vi "SCTL Sector Accumulation.vi"() -> (2 "Accummulated":T1(array[cluster]), 3 "New Data?":bool)   [LabVIEW 2013]
uses:
  Accumulated Count Array Fixed Point.ctl
  <vilib>/rvi/FIFO/Fifo_Resource/nirvififoEmulationReadFpgaImpl.vi
  <vilib>/rvi/DataTransferAndStorage/Container/Common/niFpgaContainerGetUniqueNameForEmu.vi
  <vilib>/rvi/Memory/Memory_Emulation/nirvimemoryFastEmulationFpgaImpl.vi
  <instcachedir>/0/nirvimemoryFastEmulationFpgaImpl_5FBAB50466BC4C939F684F8805638BFC.lvgen/nirvimemoryFastEmulationFpgaImpl_5FBAB50466BC4C939F684F8805638BFC_012.vi
  <vilib>/rvi/Memory/Memory_Emulation/nirvimemoryFastEmulation.vi
  <vilib>/rvi/Memory/Memory_Emulation/nirvimemoryEmulation.vi
  <vilib>/rvi/DataTransferAndStorage/Container/XNode/niFpgaContainer.xnode
  <vilib>/rvi/FIFO/Fifo_Resource/nirvififoEmulationRead.vi
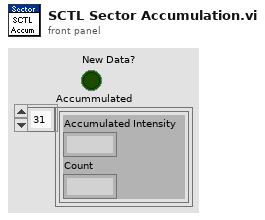
[diagram p1: front panel]
types:
  T1 = cluster{"Accumulated Intensity":fxp<+,20,20>, "Count":fxp<+,12,12>}[]
  T2 = cluster{"Accumulated Intensity":fxp<+,8,8>, "Count":fxp<+,1,1>}
  T3 = typedef "Accumulated Count Array Fixed Point.ctl" = cluster{"Accumulated Intensity":fxp<+,20,20>, "Count":fxp<+,12,12>}[]
  T4 = cluster{"Accumulated Intensity":fxp<+,21,21>, "Count":fxp<+,13,13>}[]
  T5 = cluster{"Accumulated Intensity":fxp<+,22,22>, "Count":fxp<+,14,14>}[]
  T6 = cluster{"Accumulated Intensity":fxp<+,23,23>, "Count":fxp<+,15,15>}[]
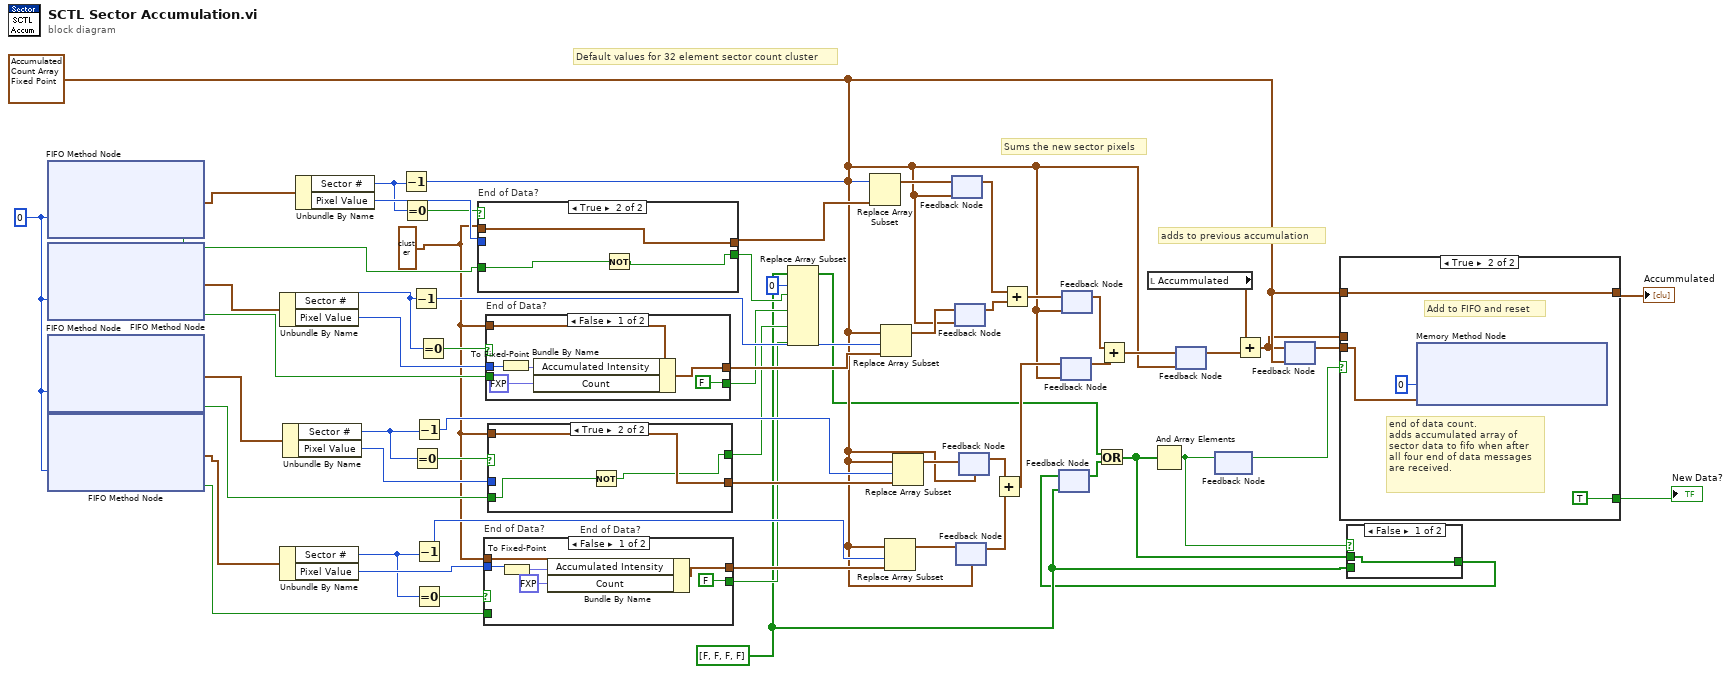
[diagram p0: block diagram]
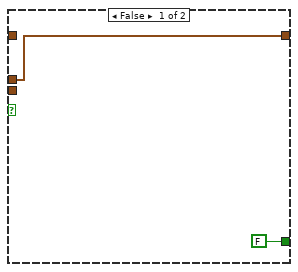
[diagram p3: hidden frame]
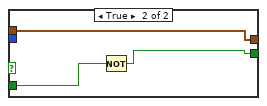
[diagram p4: hidden frame]
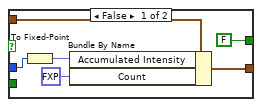
[diagram p5: hidden frame]
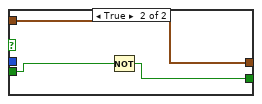
[diagram p6: hidden frame]
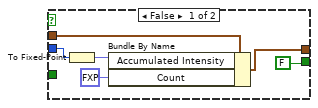
[diagram p7: hidden frame]
diagram:
  w5 = 0 ("Timeout")
  w7 = bool[] [FALSE, FALSE, FALSE, FALSE]
  w37 = T2 {"Accumulated Intensity"=0.0, "Count"=0.0} ("Accumulated Sector Cluster")
  w19 = T3 [{"Accumulated Intensity"=0.0, "Count"=0.0}, {"Accumulated Intensity"=0.0, "Count"=0.0}, {"Accumulated Intensity"=0.0, "Count"=0.0}, {"Accumulated Intensity"=0.0, "Count"=0.0}, {"Accumulated Intensity"=0.0, "Count"=0.0}, {"Accumulated Intensity"=0.0, "Count"=0.0}, {"Accumulated Intensity"=0.0, "Count"=0.0}, {"Accumulated Intensity"=0.0, "Count"=0.0}, {"Accumulated Intensity"=0.0, "Count"=0.0}, {"Accumulated Intensity"=0.0, "Count"=0.0}, {"Accumulated Intensity"=0.0, "Count"=0.0}, {"Accumulated Intensity"=0.0, "Count"=0.0}, {"Accumulated Intensity"=0.0, "Count"=0.0}, {"Accumulated Intensity"=0.0, "Count"=0.0}, {"Accumulated Intensity"=0.0, "Count"=0.0}, {"Accumulated Intensity"=0.0, "Count"=0.0}, {"Accumulated Intensity"=0.0, "Count"=0.0}, {"Accumulated Intensity"=0.0, "Count"=0.0}, {"Accumulated Intensity"=0.0, "Count"=0.0}, {"Accumulated Intensity"=0.0, "Count"=0.0}, {"Accumulated Intensity"=0.0, "Count"=0.0}, {"Accumulated Intensity"=0.0, "Count"=0.0}, {"Accumulated Intensity"=0.0, "Count"=0.0}, {"Accumulated Intensity"=0.0, "Count"=0.0}, {"Accumulated Intensity"=0.0, "Count"=0.0}, {"Accumulated Intensity"=0.0, "Count"=0.0}, {"Accumulated Intensity"=0.0, "Count"=0.0}, {"Accumulated Intensity"=0.0, "Count"=0.0}, {"Accumulated Intensity"=0.0, "Count"=0.0}, {"Accumulated Intensity"=0.0, "Count"=0.0}, {"Accumulated Intensity"=0.0, "Count"=0.0}, {"Accumulated Intensity"=0.0, "Count"=0.0}] ("Test Accumulated Array")
  # "adds to previous accumulation"
  # "Sums the new sector pixels"
  # "Default values for 32 element sector count cluster"
  n1 = xnode ("FIFO Method Node")("Timeout"=w5) -> ("Element"=w4:cluster{"Sector #":u8, "Pixel Value":u8}, "Timed Out?"=w41:bool)  [unwired: 1 in, 1 out]
  n2 = xnode ("FIFO Method Node")("Timeout"=w5) -> ("Element"=w3:cluster{"Sector #":u8, "Pixel Value":u8}, "Timed Out?"=w40:bool)  [unwired: 1 in, 1 out]
  n3 = xnode ("FIFO Method Node")("Timeout"=w5) -> ("Element"=w2:cluster{"Sector #":u8, "Pixel Value":u8}, "Timed Out?"=w39:bool)  [unwired: 1 in, 1 out]
  n4 = xnode ("FIFO Method Node")("Timeout"=w5) -> ("Element"=w1:cluster{"Sector #":u8, "Pixel Value":u8}, "Timed Out?"=w38:bool)  [unwired: 1 in, 1 out]
  n5 = Unbundle By Name(w3) -> ("Sector #"=w49:u8, "Pixel Value"=w59:u8)
  n6 = Unbundle By Name(w1) -> ("Sector #"=w45:u8, "Pixel Value"=w53:u8)
  n7 = Unbundle By Name(w2) -> ("Sector #"=w47:u8, "Pixel Value"=w56:u8)
  n8 = Unbundle By Name(w4) -> ("Sector #"=w51:u8, "Pixel Value"=w61:u8)
  n9 = Decrement(x=w51) -> (x-1=w62:u8)
  n10 = Equal To 0?(x=w51) -> (x = 0?=w50:bool)
  n11 = Decrement(x=w49) -> (x-1=w58:u8)
  n12 = Equal To 0?(x=w47) -> (x = 0?=w46:bool)
  n13 = Decrement(x=w47) -> (x-1=w42:u8)
  n14 = Decrement(x=w45) -> (x-1=w55:u8)
  n15 = Equal To 0?(x=w45) -> (x = 0?=w44:bool)
  n16 = Equal To 0?(x=w49) -> (x = 0?=w48:bool)
  n17 = case "End of Data?" shown="True" w50 {
    tunnel: w61 -> [w65 _]
    tunnel: [w68 w71] -> w60
    tunnel: w37 -> [w67 w71]
    tunnel: [FALSE w69] -> w15
    tunnel: w41 -> [_ w70]
    frame False {
      n18 = To Fixed-Point(number=w65) -> (fixed-point=w64:fxp<+,8,8>)  [unwired: 1 in]
      n19 = Bundle By Name(cluster=w67, "Accumulated Intensity"=w64, "Count"=fxp<+,1,1> 1.0) -> (w68:T2)
    }
    frame True {
      n20 = Not(x=w70) -> (.not. x?=w69:bool)
    }
  }
  n21 = case "End of Data?" shown="False" w44 {
    tunnel: [w77 w80] -> w54
    tunnel: w37 -> [w76 w80]
    tunnel: w53 -> [w73 _]
    tunnel: [FALSE w78] -> w12
    tunnel: w38 -> [_ w79]
    frame False {
      n22 = To Fixed-Point(number=w73) -> (fixed-point=w74:fxp<+,8,8>)  [unwired: 1 in]
      n23 = Bundle By Name(cluster=w76, "Accumulated Intensity"=w74, "Count"=fxp<+,1,1> 1.0) -> (w77:T2)
    }
    frame True {
      n24 = Not(x=w79) -> (.not. x?=w78:bool)
    }
  }
  n25 = case "End of Data?" shown="False" w48 {
    tunnel: w59 -> [w83 _]
    tunnel: w37 -> [w86 w89]
    tunnel: [w85 w89] -> w52
    tunnel: [FALSE w87] -> w14
    tunnel: w40 -> [_ w88]
    frame False {
      n26 = To Fixed-Point(number=w83) -> (fixed-point=w82:fxp<+,8,8>)  [unwired: 1 in]
      n27 = Bundle By Name(cluster=w86, "Accumulated Intensity"=w82, "Count"=fxp<+,1,1> 1.0) -> (w85:T2)
    }
    frame True {
      n28 = Not(x=w88) -> (.not. x?=w87:bool)
    }
  }
  n29 = case "End of Data?" shown="True" w46 {
    tunnel: [w95 w98] -> w57
    tunnel: w56 -> [w92 _]
    tunnel: w37 -> [w94 w98]
    tunnel: [FALSE w96] -> w13
    tunnel: w39 -> [_ w97]
    frame False {
      n30 = To Fixed-Point(number=w92) -> (fixed-point=w91:fxp<+,8,8>)  [unwired: 1 in]
      n31 = Bundle By Name(cluster=w94, "Accumulated Intensity"=w91, "Count"=fxp<+,1,1> 1.0) -> (w95:T2)
    }
    frame True {
      n32 = Not(x=w97) -> (.not. x?=w96:bool)
    }
  }
  n33 = Replace Array Subset(array=w7, new element #1=w15, index #1=0 ("index"), new element #2=w14, new element #3=w13, new element #4=w12) -> (w11:bool[])  [unwired: 3 in]
  n34 = Replace Array Subset(array=w19, new element=w60, index=w62) -> (w34:T3)
  n35 = Replace Array Subset(array=w19, new element=w52, index=w58) -> (w32:T3)
  n36 = Replace Array Subset(array=w19, new element=w54, index=w55) -> (w28:T3)
  n37 = Replace Array Subset(array=w19, new element=w57, index=w42) -> (w30:T3)
  n38 = feedback #1(w19) -> (w33:T3)
  n39 = feedback-in #1(w34) -> ()
  n40 = feedback #2(w19) -> (w31:T3)
  n41 = feedback-in #2(w32) -> ()
  n42 = feedback #3(w19) -> (w27:T3)
  n43 = feedback-in #3(w28) -> ()
  n44 = feedback #4(w19) -> (w29:T3)
  n45 = feedback-in #4(w30) -> ()
  n46 = Add(x=w29, y=w27) -> (x+y=w24:T4)
  n47 = Add(x=w33, y=w31) -> (x+y=w26:T4)
  n48 = feedback #5(w7) -> (w17:bool[])
  n49 = feedback #6(w19) -> (w23:T4)
  n50 = feedback-in #6(w24) -> ()
  n51 = feedback #7(w19) -> (w25:T4)
  n52 = feedback-in #7(w26) -> ()
  n53 = Or(x=w11, y=w17) -> (x .or. y?=w8:bool[])
  n54 = Add(x=w25, y=w23) -> (x+y=w22:T5)
  n55 = local read "Accummulated"() -> (w36:T1)
  n56 = And Array Elements(Boolean array=w8) -> (logical AND=w9:bool)
  n57 = feedback #8(w19) -> (w21:T5)
  n58 = feedback-in #8(w22) -> ()
  n59 = feedback #9() -> (w10:bool)  [unwired: 1 in]
  n60 = feedback-in #9(w9) -> ()
  n61 = Add(x=w36, y=w21) -> (x+y=w18:T6)
  n62 = feedback #10(w19) -> (w20:T6)
  n63 = feedback-in #10(w18) -> ()
  n64 = case shown="True" w10 {
    tunnel: w20 -> [_ w101]
    tunnel: w19 -> [_ w102]
    tunnel: [FALSE ("New Data?") TRUE ("New Data?")] -> w43
    tunnel: [w99 w102] -> w35
    tunnel: w18 -> [w99 _]
    frame False {
    }
    frame True {
      # "end of data count.\nadds accumulated array of\nsector data to fifo when after\nall four end of data messages\nare received."
      # "Add to FIFO and reset"
      n65 = xnode ("Memory Method Node")("Address"=u32 0, "Data"=w101) -> ()  [unwired: 1 in, 1 out]
    }
  }
  "New Data?" <- w43
  "Accummulated" <- w35
  n66 = case shown="False" w9 {
    tunnel: w8 -> [w105 _]
    tunnel: w7 -> [_ w106]
    tunnel: [w105 w106] -> w6
    frame False {
    }
    frame True {
    }
  }
  n67 = feedback-in #5(w6) -> ()
